vi "PrintResults.vi"(0 "Prime_Sieve in":refnum<class "Prime_Sieve.lvclass">, 5 "Duration":dbl, 7 "Passes":i32, 11 "error in (no error)":errorcluster) -> (4 "Prime_Sieve out":refnum<class "Prime_Sieve.lvclass">, 8 "Result":string, 15 "error out":errorcluster)   [LabVIEW 2025, in "Prime_Sieve.lvclass"]
uses:
  Prime_Sieve.lvclass
  Prime_Sieve.lvclass/Prime_Sieve.ctl
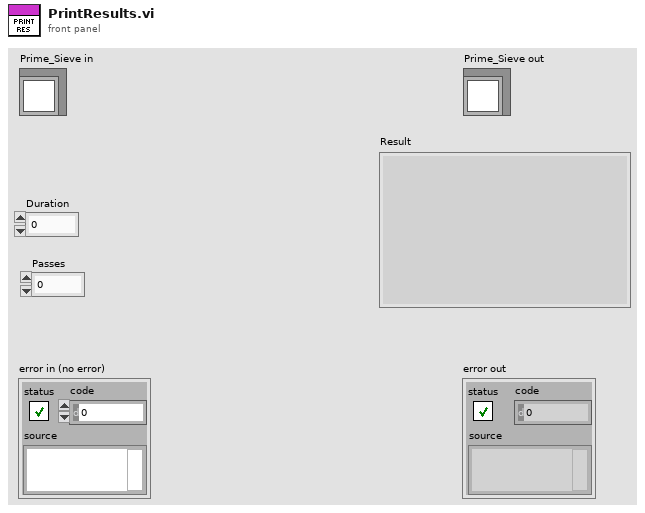
[diagram p1: front panel]
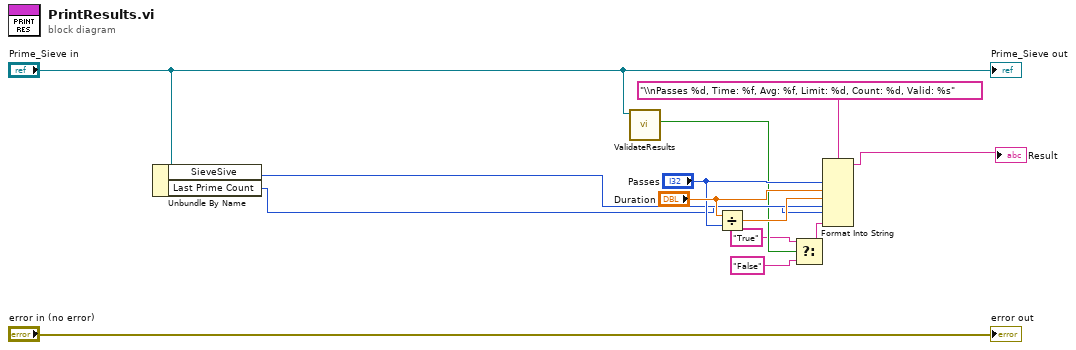
[diagram p0: block diagram]
diagram:
  n1 = Unbundle By Name("Prime_Sieve in") -> ("SieveSive"=w6:i32, "Last Prime Count"=w1:i32)
  n2 = call "ValidateResults.vi"("Prime_Sieve in"="Prime_Sieve in") -> ("Valid Results?"=w5:bool)  [unwired: 8 in, 2 out]
  n3 = Divide(x="Duration", y="Passes") -> (x/y=w7:dbl)
  n4 = Select(t="True", s=w5, f="False") -> (s? t:f=w2:string)
  n5 = Format Into String(format string="\\nPasses %d, Time: %f, Avg: %f, Limit: %d, Count: %d, Valid: %s", "Passes", "Duration", w7, w6, w1, w2) -> (resulting string=→"Result":string)  [unwired: 2 in, 1 out]
  "error out" <- "error in (no error)"
  "Prime_Sieve out" <- "Prime_Sieve in"
